vi "UI (Beginner).vi"() -> ()   [LabVIEW 2017, in "UI.lvlib"]
doc: "The Queued Message Handler of a Worker."
uses:
  UI.lvlib
  _support/UI State.ctl
  1af51285-6659-428e-9c15-de70f1a207c9.vi
  1756710f-d813-4077-a3f9-6f06171a4225.vi
  b1498353-a107-4479-98d0-7e76c0451ff6.vi
  242d01f8-d211-4c25-bb6c-8191a2acbe42.vi
  <userlib>/_NEVSTOP/Communicable State Machine(CSM)/AdvanceAPI/CSM - Revert Arguments-Safe String.vi
  <userlib>/_NEVSTOP/Communicable State Machine(CSM)/_Shared/Trim Single-line Text.vi
  <userlib>/_NEVSTOP/Communicable State Machine(CSM)/AdvanceAPI/CSM - Make String Arguments Safe.vi
  <userlib>/_NEVSTOP/Communicable State Machine(CSM)/AdvanceAPI/CSM - Break Down Multiple States String.vi
  <userlib>/_NEVSTOP/Communicable State Machine(CSM)/AdvanceAPI/CSM - Keywords.vi
  <userlib>/_NEVSTOP/Communicable State Machine(CSM)/addons/INI-Static-Variable-Support/_Support/instances/_CSM - Read File Logger Configuration - v1.0.vi
  <userlib>/_NEVSTOP/Communicable State Machine(CSM)/addons/API-String-Arugments-Support/_Support/Convert API String Arguments to Data(variant).vi
  <userlib>/_NEVSTOP/Communicable State Machine(CSM)/addons/API-String-Arugments-Support/_Support/Query Data as API String Arguments(variant).vi
  <userlib>/_NEVSTOP/Communicable State Machine(CSM)/addons/MassData-Parameter/_support/FGV-MassData(lvlibp).vi
  <userlib>/_NEVSTOP/Communicable State Machine(CSM)/_Polymophic/Add State(s) to Queue By BOOL(Element).vi
  Acquisition/Acquisition.lvlib
  Logging/Logging.lvlib
  <userlib>/_NEVSTOP/Communicable State Machine(CSM)/Communicable State Machine.lvlib
  <userlib>/_NEVSTOP/Communicable State Machine(CSM)/addons/MassData-Parameter/CSM MassData Parameter Support.lvlib
  <userlib>/_NEVSTOP/Communicable State Machine(CSM)/addons/INI-Static-Variable-Support/INI-Static-Variable-Support.lvlib
  <userlib>/_NEVSTOP/Communicable State Machine(CSM)/addons/Logger/CSM File Logger.lvlib
  <userlib>/_NEVSTOP/Communicable State Machine(CSM)/addons/Watchdog/CSM Watchdog.lvlib
  <userlib>/_NEVSTOP/Communicable State Machine(CSM)/_Polymophic/Build Synchronous Message with Arguments.vi
panel:
  out "WaveformGraph":waveform(dbl)[](graph)
  in  "Settings":bool
  in  "Start":bool
  in  "Stop":bool
  out "Status":string
  in  "Exit":bool
  # "Continuous Measurement and Data Logger - CSM Version"
  # "Beginner Example"
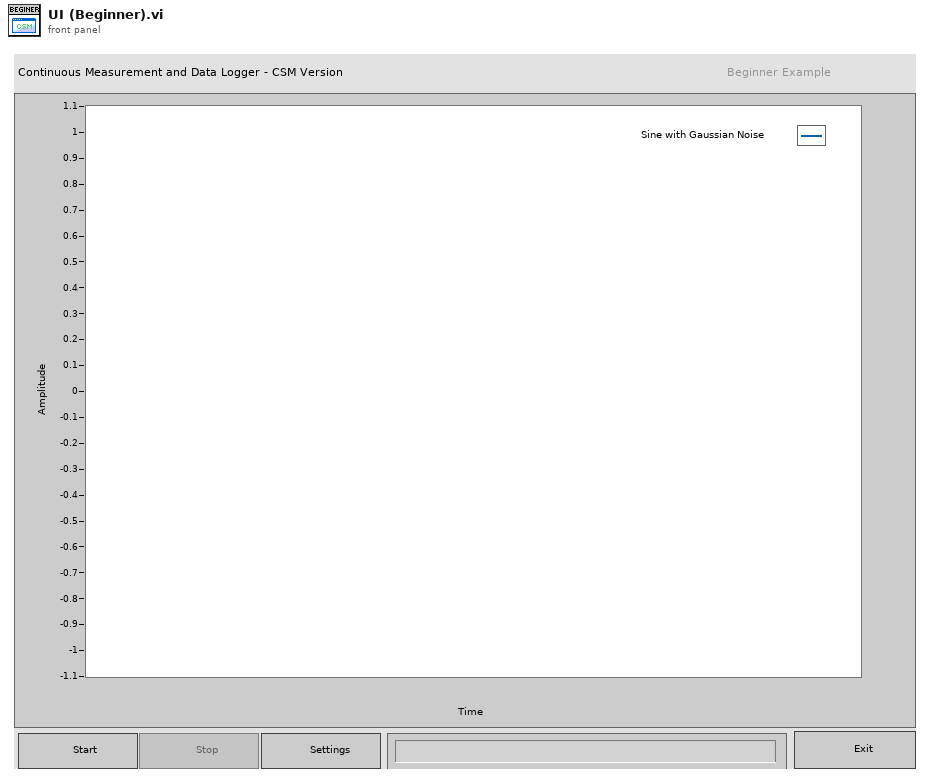
[diagram p1: front panel]
types:
  T1 = cluster{"Enable":bool, "Limit":cluster{"FileSize":i64, "FileNum":i32}, "Timestamp.Format":string, "AutoExit":bool}
  T2 = enum32{"Invalid", "Standard", "Closed", "Hidden", "Minimized", "Maximized"}
  T3 = enum32{"invalid app kind", "Development System", "Run Time System", "Student Edition", "Embedded LabVIEW", "Evaluation", "Custom"}
  T4 = typedef "UI.lvlib/UI State.ctl" = enum16{"Idle", "Acquiring and Logging", "Waiting for Exit", "Waiting for Exit (Acq Stopped)", "Waiting for Exit (Log Stopped)", "Waiting for Stop", "Waiting for Stop (Acq Stopped)", "Waiting for Stop (Log Stopped)"}
  T5 = enum32{"Invalid", "Default", "Floating", "Floating/Auto-Hide", "Modal"}
  T6 = typedef "Communicable State Machine.lvlib/_CSM_Response Source Message.ctl" = cluster{"‘State":string, "’Arguments":string, "’Error":errorcluster}
  T7 = cluster{"Current VI Reference":refnum<vi>, "Close Panel on Exit?":bool}
  T8 = cluster{"Core":cluster{"Current VI Reference":refnum<vi>, "Close Panel on Exit?":bool}, "UI Refs":cluster{"Start Ref":refnum<vi>, "Stop Ref":refnum<vi>, "Settings Ref":refnum<vi>, "Exit Ref":refnum<vi>, "Status Ref":refnum<vi>, "Data Ref":refnum<vi>, "Data Source Ref":refnum<vi>}, "State":T4, "Relationships":string}
  T9 = cluster{"Start Ref":refnum<vi>, "Stop Ref":refnum<vi>, "Settings Ref":refnum<vi>, "Exit Ref":refnum<vi>, "Status Ref":refnum<vi>, "Data Ref":refnum<vi>, "Data Source Ref":refnum<vi>}
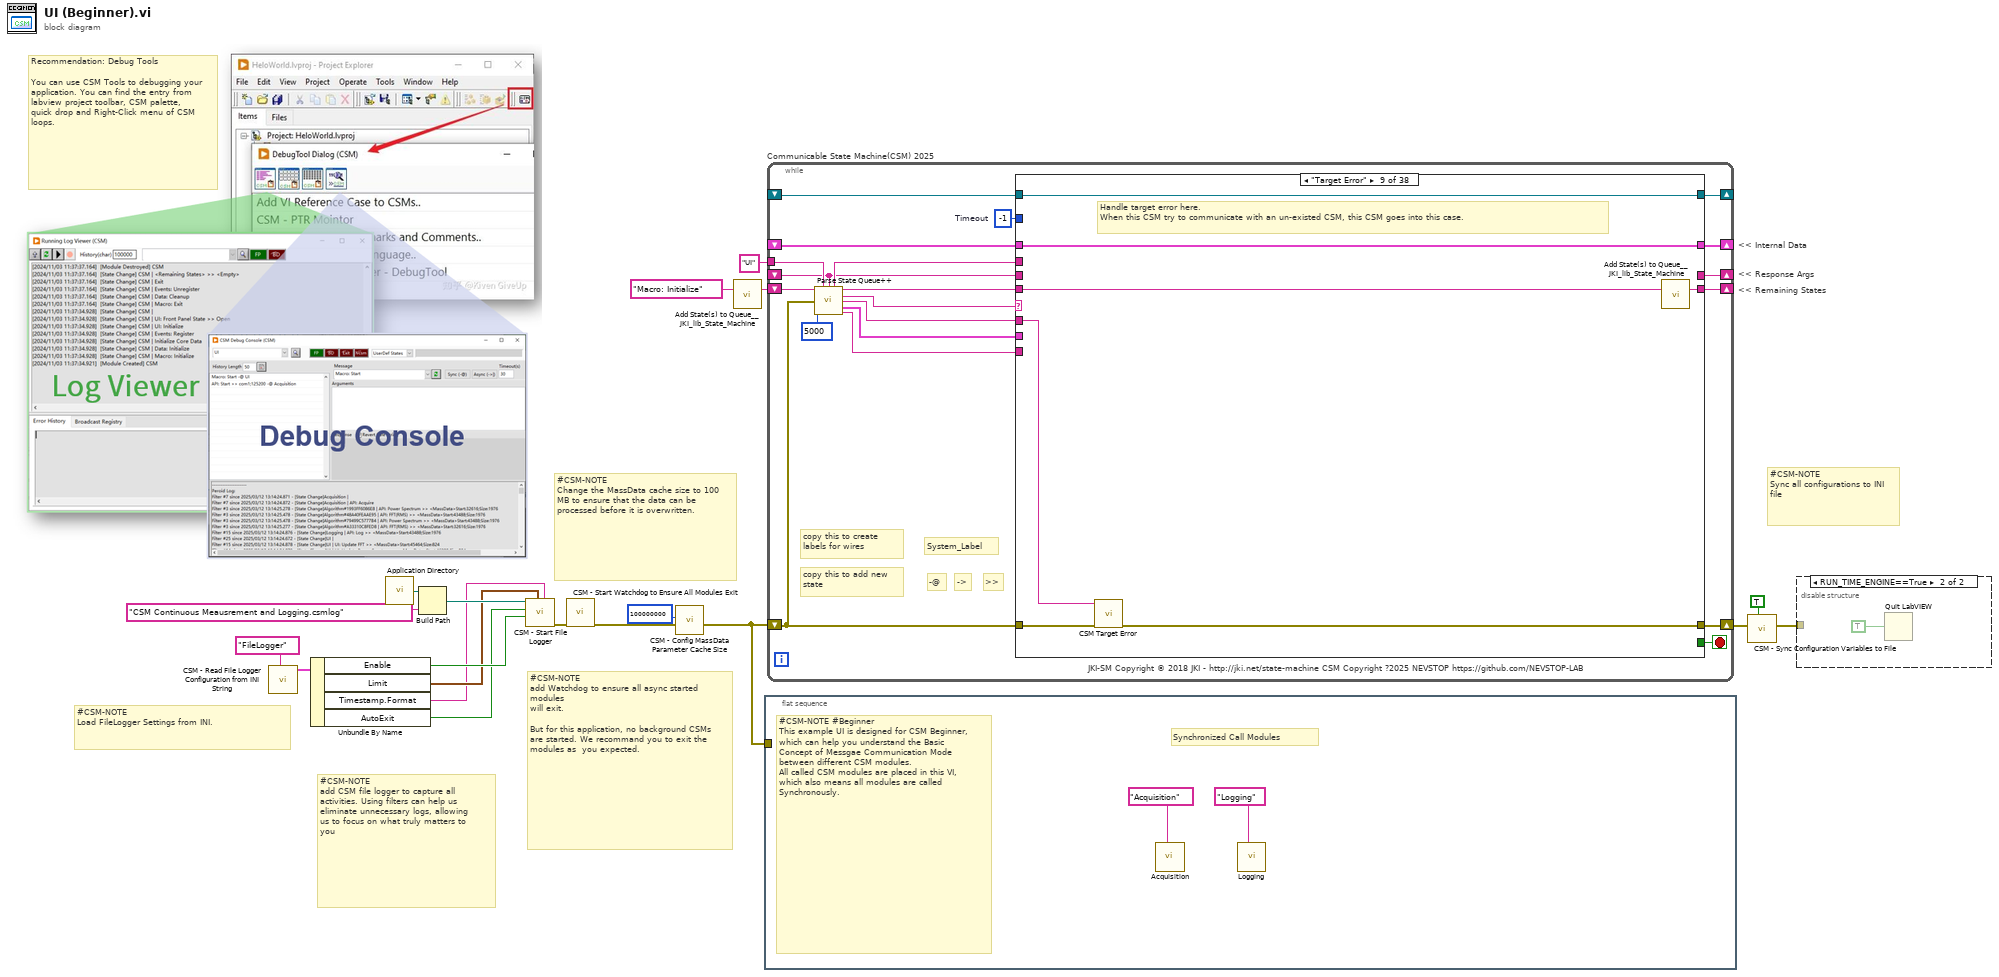
[diagram p0: block diagram]
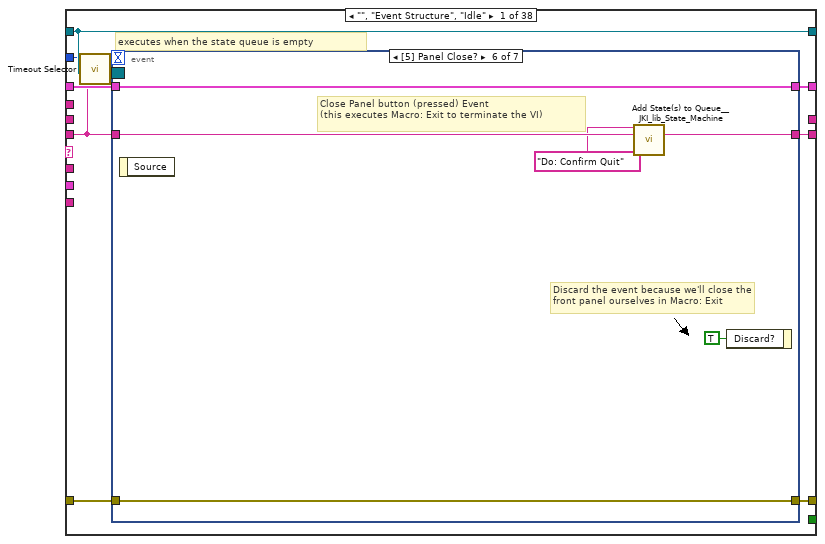
[diagram p3: hidden frame]
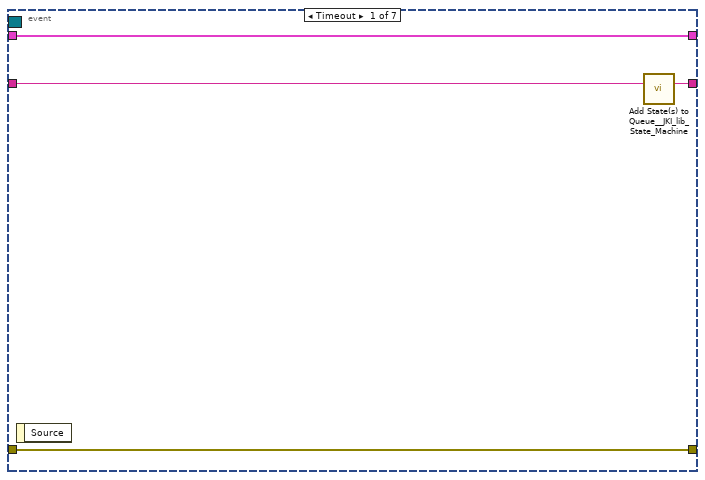
[diagram p4: hidden frame]
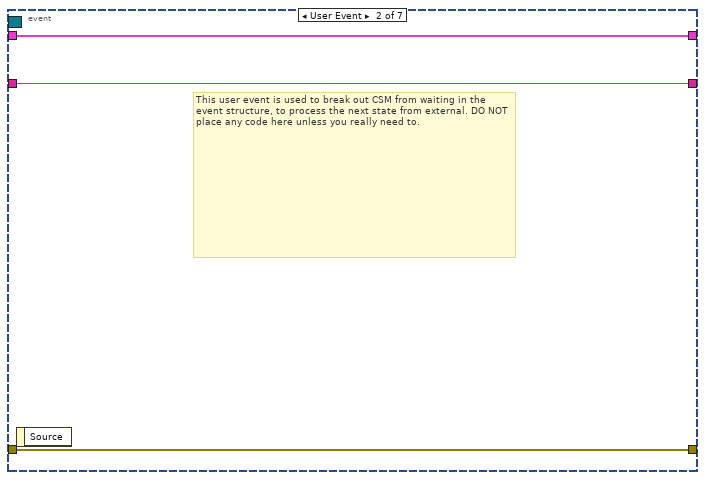
[diagram p5: hidden frame]
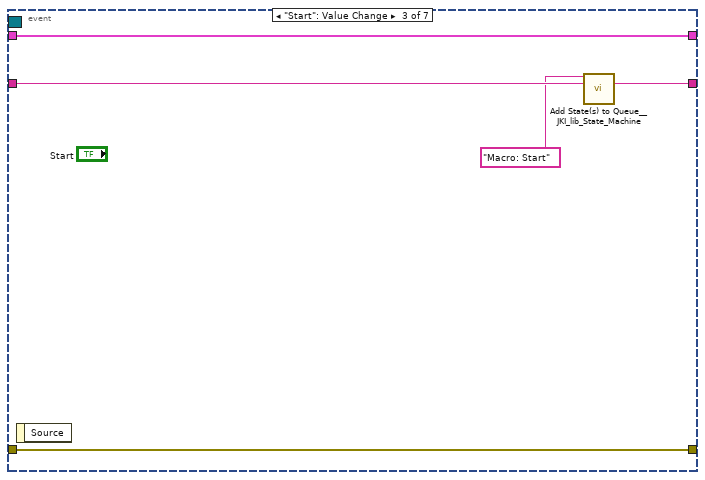
[diagram p6: hidden frame]
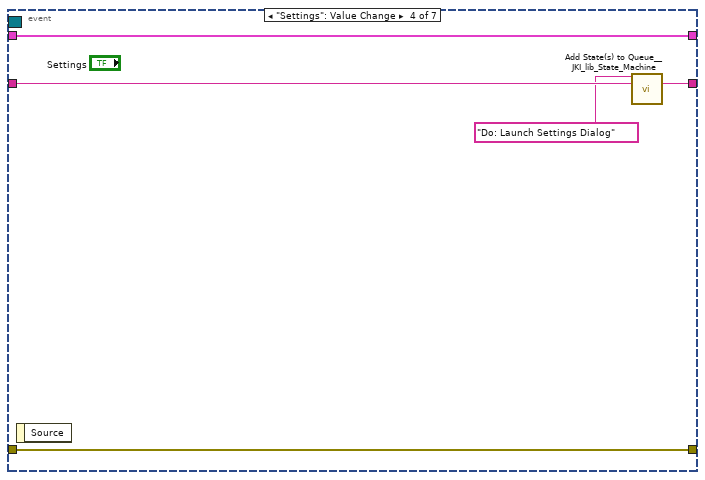
[diagram p7: hidden frame]
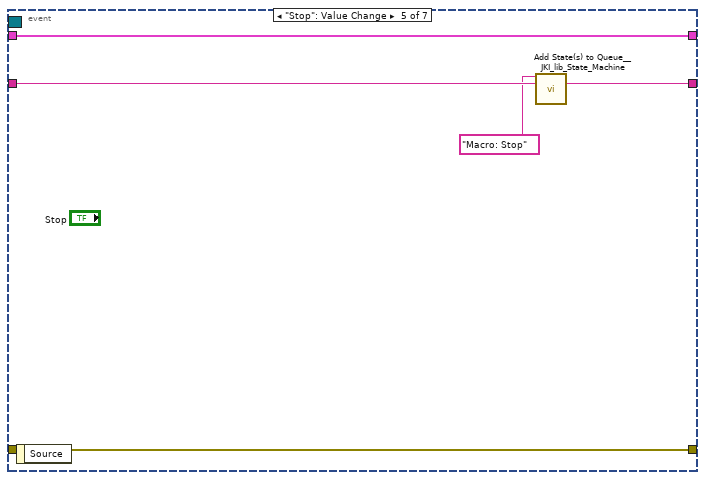
[diagram p8: hidden frame]
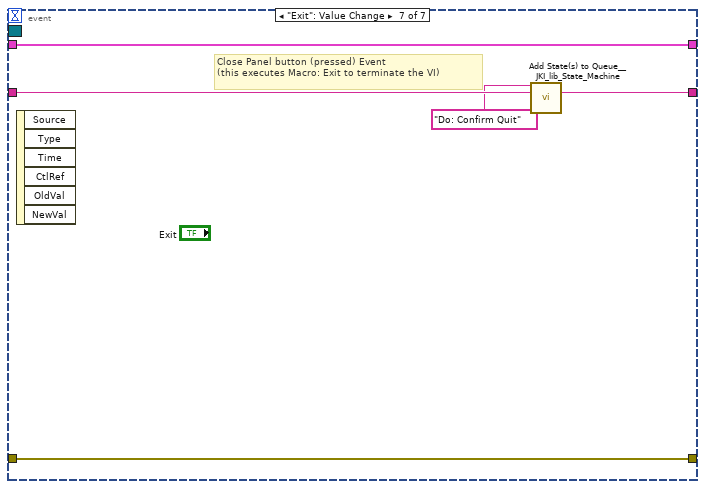
[diagram p9: hidden frame]
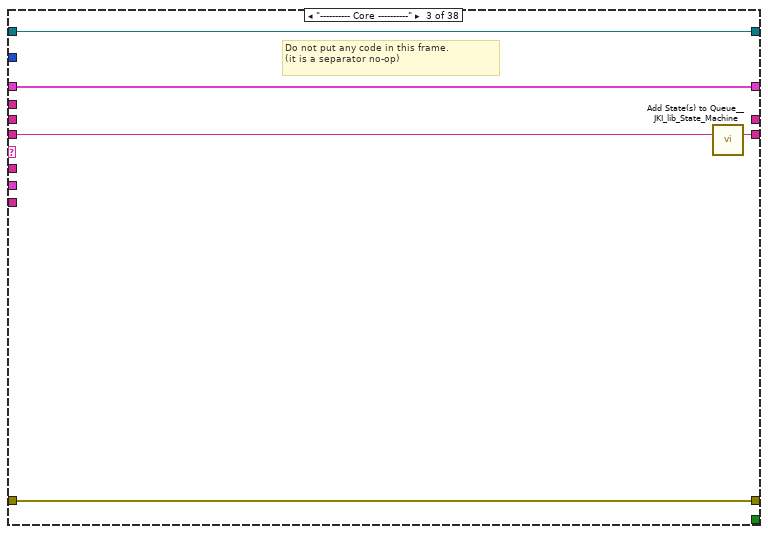
[diagram p11: hidden frame]
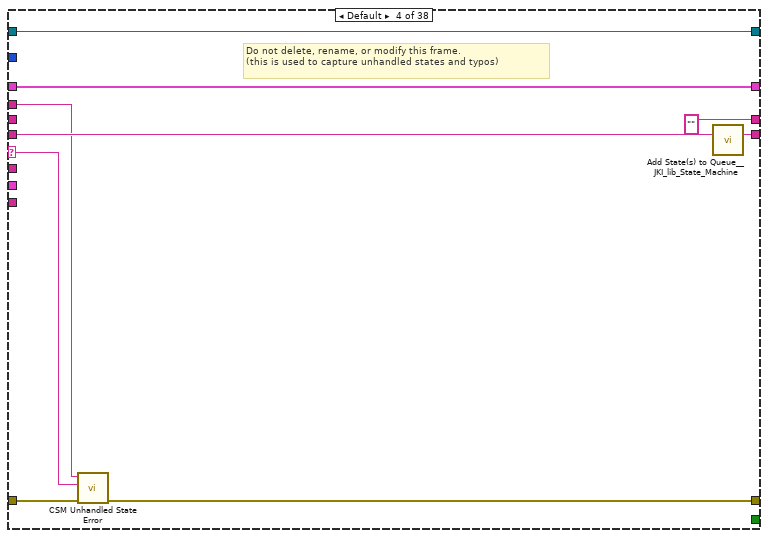
[diagram p12: hidden frame]
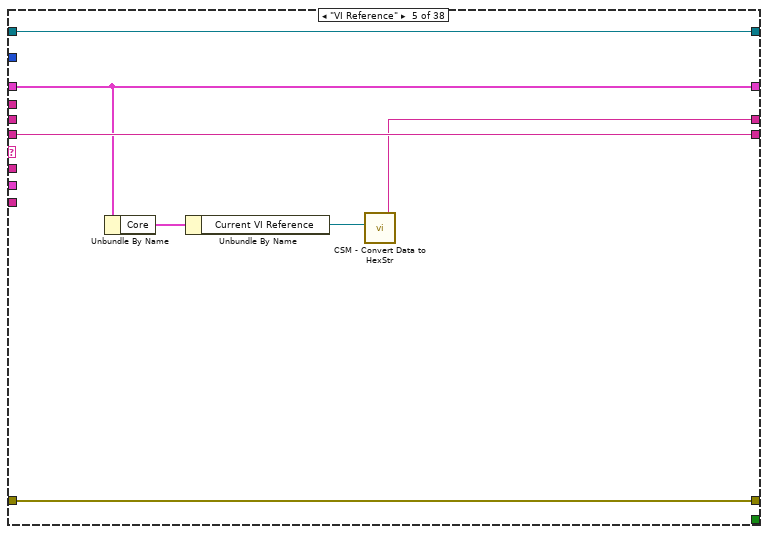
[diagram p13: hidden frame]
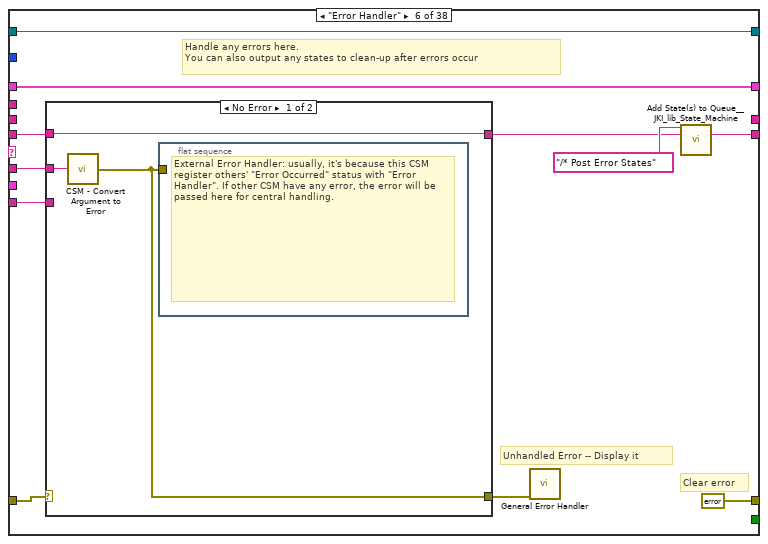
[diagram p14: hidden frame]
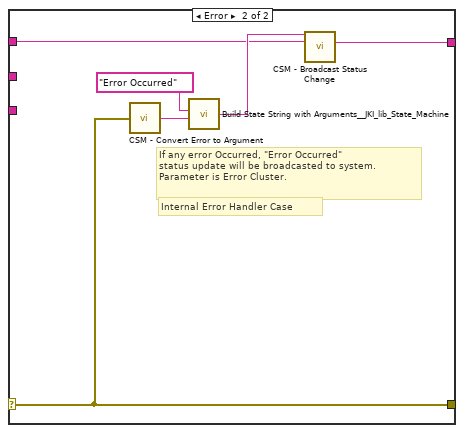
[diagram p15: hidden frame]
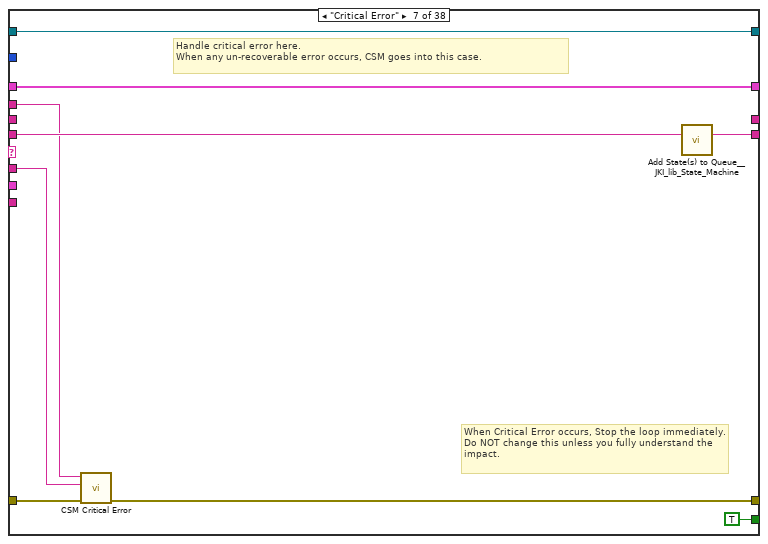
[diagram p16: hidden frame]
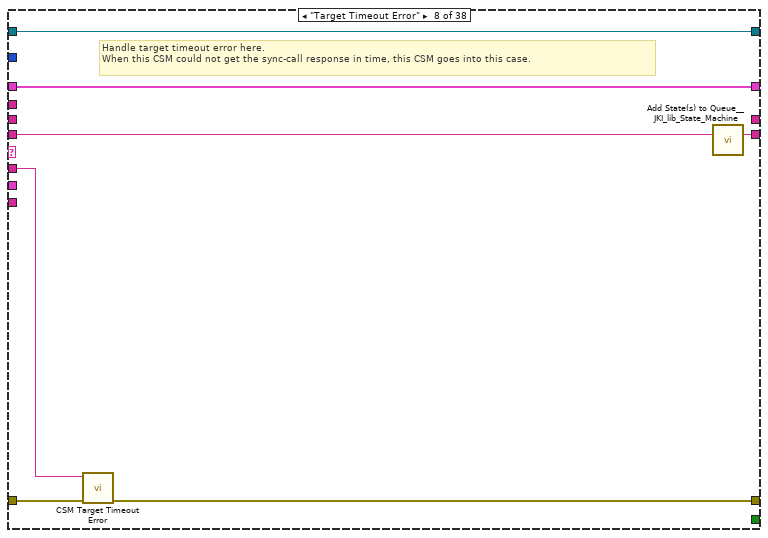
[diagram p17: hidden frame]
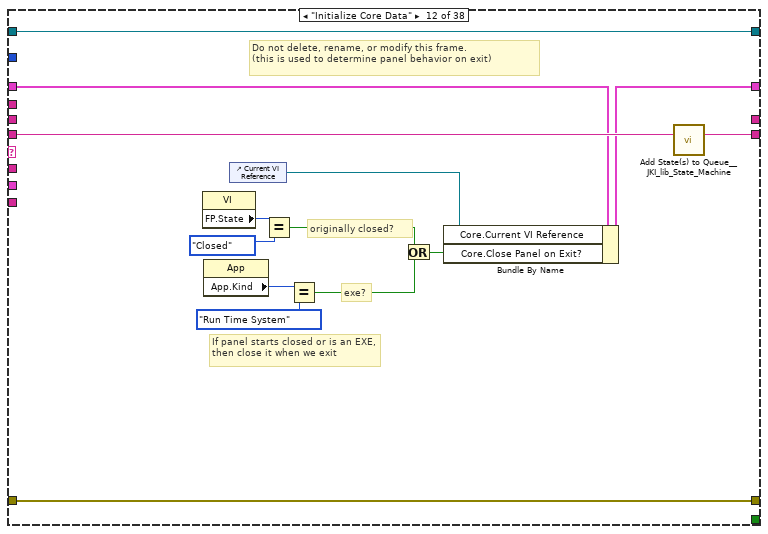
[diagram p20: hidden frame]
diagram:
  # "#CSM-NOTE\nSync all configurations to INI file"
  # "#CSM-NOTE\nChange the MassData cache size to 100 MB to ensure that the data can be processed before it is overwritten."
  # "Recommendation: Debug Tools\n\nYou can use CSM Tools to debugging your application. You can find the entry from labview project toolbar, CSM palette, quick drop and Right-Click menu of CSM loops."
  # "#CSM-NOTE\nLoad FileLogger Settings from INI."
  # "#CSM-NOTE\nadd CSM file logger to capture all activities. Using filters can help us eliminate unnecessary logs, allowing us to focus on what truly matters to you"
  # "#CSM-NOTE\nadd Watchdog to ensure all async started modules\nwill exit. \n\nBut for this application, no background CSMs are started. We recommand you to exit the modules as  you expected."
  # "<< Internal Data"
  # "<< Response Args"
  # "<< Remaining States"
  n1 = call-poly <userlib>:"CSM - Read File Logger Configuration from INI String.vi"("Section Name(\"FileLogger\")"="FileLogger" ("Section Name(\"\" as Default)")) -> ("FileLogger Configuration-v1"=w11:T1)  [unwired: 7 in, 1 out]
  n2 = Unbundle By Name(w11) -> ("Enable"=w10:bool, "Limit"=w9:cluster{"FileSize":i64, "FileNum":i32}, "Timestamp.Format"=w7:string, "AutoExit"=w8:bool)
  n3 = call <vilib>:"Application Directory.vi"() -> ("Application Directory"=w16:path)
  n4 = Build Path(base path=w16, name or relative path="CSM Continuous Meausrement and Logging.csmlog") -> (appended path=w14:path)
  n5 = call <userlib>:"CSM - Start File Logger.vi"("Timestamp Format"=w7, "Log Limit"=w9, "Watchdog? (T)"=w10, "Exit When All Module Exist? (F)"=w8, "Log File Path"=w14) -> ("error out"=w13:errorcluster)  [unwired: 4 in, 2 out]
  n6 = call <userlib>:"CSM - Start Watchdog to Ensure All Modules Exit.vi"("error in (no error)"=w13) -> ("error out"=w5:errorcluster)  [unwired: 10 in]
  n7 = call <userlib>:"CSM - Config MassData Parameter Cache Size.vi"("Error in"=w5, "Size (50M)"=100000000 ("size(1M)")) -> ("Error out"=w4:errorcluster)  [unwired: 9 in]
  n8 = call <vilib>:"Add State(s) to Queue__JKI_lib_State_Machine.vi"("State(s) in (\"\")"="Macro: Initialize") -> ("States Out"=w17:string)  [unwired: 14 in]
  n9 = flat-sequence {
    tunnel: w4 -> [_]
    frame #0 {
      # "Synchronized Call Modules"
      # "#CSM-NOTE #Beginner\nThis example UI is designed for CSM Beginner, which can help you understand the Basic Concept of Messgae Communication Mode between different CSM modules.\nAll called CSM modules are placed in this VI, which also means all modules are called  Synchronously."
      n10 = call "Acquisition.vi"("Name(\"\" to use uuid)"="Acquisition" ("Name(\"\" to use uuid)")) -> ()  [unwired: 11 in]
      n11 = call "Logging.vi"("Name(\"\" to use uuid)"="Logging" ("Name(\"\" to use uuid)")) -> ()  [unwired: 11 in]
    }
  }
  n12 = while "Communicable State Machine(CSM) 2025" {
    shift-right: [w36] -> _
    shift-left: _ -> [w35]
    shift-right: [w39] -> w2
    shift-left: w4 -> [w33]
    shift-right: [w38] -> _
    shift-left: w17 -> [w40]
    tunnel: "UI" ("Name(\"\" to use uuid)") -> [w28]
    shift-right: [w31] -> _
    shift-left: _ -> [w23]
    shift-right: [w30] -> _
    shift-left: _ -> [w29]
    stop <- w37 stop-if-true
    w34 = -1  # Timeout
    # "JKI-SM Copyright © 2018 JKI - http://jki.net/state-machine CSM Copyright ?2025 NEVSTOP https://github.com/NEVSTOP-LAB"
    # "copy this to add new state"
    # ">>"
    # "->"
    # "-@"
    # "copy this to create labels for wires"
    # "System_Label"
    n13 = call <userlib>:"Parse State Queue++.vi"("State Queue"=w40, "Name (\"\" to Use UUID)"=w28, "Response Arguments"=w23, "Previous Error"=w33, "Response Timeout (-2 Use Global Settings)"=5000 ("Response Timeout(1000ms)")) -> ("Name Used"=w24:string, "Remaining States"=w41:string, "Current State"=w27:string, "Arguments"=w22:string, "Additional Information"=w26:T6, "Source CSM"=w25:string)  [unwired: 5 in]
    n14 = case shown="\"Target Error\"" w27 {
      selector: w27 -> [_ _ _ w95 _ _ _ _ _ _ _ _ _ _ _ _ _ _ _ _ _ _ _ _ _ _ _ _ _ _ _ _ _ _ _ _ _ _]
      tunnel: w41 -> [w42 w86 w92 w100 w107 w112 w135 w143 w150 w154 w158 w173 w180 w185 w194 w200 w207 w214 w219 w225 w229 w235 w252 w265 w278 w286 w302 w376 w385 w396 w403 w405 w416 w434 w459 w465 w473 w511]
      tunnel: w22 -> [_ _ _ _ _ w110 w129 w139 w146 _ _ _ _ _ _ w198 w204 _ _ _ _ _ _ _ _ w281 w296 w371 w389 _ _ _ _ _ _ w460 _ _]
      tunnel: w35 -> [w49 w85 w89 w98 w106 w118 w136 w141 w148 w153 w157 w166 w178 w182 _ w197 w205 w209 w216 w224 w228 w232 w239 w255 w268 w284 w298 w374 w391 w393 w400 w408 w412 w432 w456 w462 w466 w506]
      tunnel: [w48 w87 w90 w94 w108 errorcluster {"status"=FALSE, "code"=0, "source"=""} ("error out") w131 w138 w145 w155 w159 w170 w177 w183 w188 w196 w203 w210 w217 w220 w227 w233 w250 w266 w279 w282 w299 w368 w387 w394 w401 w411 w420 _ w457 w463 w467 _] -> w39
      tunnel: w33 -> [w47 w87 w90 w101 w108 w116 w137 w144 w151 w155 w159 w170 w177 w183 w188 _ _ w211 w217 _ w230 w233 w250 w266 w279 w283 w300 _ _ w394 w401 w411 w420 _ w457 w463 _ _]
      tunnel: [w50 w86 w91 w99 w107 w114 w134 w142 w149 w154 w158 w172 w179 w184 w193 w200 w207 w213 w218 w225 w229 w234 w251 w265 w278 w285 w301 w376 w386 w395 w402 w406 w417 w433 w458 w464 w473 w504] -> w38
      tunnel: [_ _ _ _ _ _ TRUE _ _ _ _ _ TRUE _ _ _ _ _ _ _ _ _ _ _ _ _ _ _ _ _ _ _ _ _ _ _ _ _] -> w37
      tunnel: [w46 w85 w89 w98 w106 w118 w136 w141 w148 w153 w157 w171 w178 w182 w187 w195 w201 w209 w216 w224 w228 w232 w238 w255 w268 w284 w298 w374 w391 w393 w400 w407 w418 w432 w456 w462 w466 w505] -> w36
      tunnel: w34 -> [w44 _ _ _ _ _ _ _ _ _ _ _ _ _ _ _ _ _ _ _ _ _ _ _ _ _ _ _ _ _ _ _ _ _ _ _ _ _]
      tunnel: w25 -> [_ _ _ _ _ w109 _ _ _ _ _ _ _ _ _ _ _ _ _ _ _ _ _ _ _ _ _ _ _ _ _ _ _ _ _ _ _ _]
      tunnel: w26 -> [_ _ _ _ _ _ _ _ _ _ _ _ _ _ _ _ _ _ _ _ _ _ _ _ _ _ _ _ _ _ _ _ _ _ _ _ _ _]
      tunnel: [_ _ _ "" w102 _ _ _ _ _ _ _ _ _ _ _ w202 _ _ _ _ _ _ _ _ _ _ _ _ _ _ _ _ _ _ _ _ _] -> w31
      tunnel: [w45 w84 w88 w96 w105 w117 w132 w140 w147 w152 w156 w160 w175 w181 w191 w199 w206 w208 w215 w223 w226 w231 w249 w264 w277 w280 w295 w375 w390 w392 w399 w410 w419 w425 w455 w461 w474 w510] -> w30
      tunnel: w29 -> [w45 w84 w88 w96 w105 w117 w132 w140 w147 w152 w156 w160 w175 w181 w191 w199 w206 w208 w215 _ w226 w231 w249 w264 w277 w280 w295 w375 w390 w392 w399 w410 w419 w425 w455 w461 w474 w510]
      tunnel: w24 -> [_ _ _ w93 _ _ w130 _ _ _ _ _ _ _ _ _ _ _ _ w222 _ _ _ _ _ _ _ _ _ _ _ _ _ w423 _ _ w469 _]
      tunnel: w23 -> [_ _ _ _ _ _ _ _ _ _ _ _ _ _ _ _ _ _ _ _ _ _ _ _ _ _ _ _ _ _ _ _ _ _ _ _ _ _]
      frame "", "Event Structure", "Idle" {
        # "executes when the state queue is empty"
        n15 = call <userlib>:"Timeout Selector.vi"("Remaining States"=w42, "Timeout Expected"=w44) -> ("Timeout"=w43:i32)  [unwired: 5 in]
        n16 = event shown="[5] Panel Close?" {
          selector: w45 -> [_ _ _ _ _ _ _]
          dyn-events: _ -> [_ _ _ _ _ _ _]
          timeout: w43 -> [_ _ _ _ _ _ _]
          tunnel: w42 -> [w54 w56 w59 w64 w69 w78 w83]
          tunnel: [w53 w56 w60 w65 w70 w77 w82] -> w50
          tunnel: w49 -> [w51 w57 w61 w66 w71 w75 w80]
          tunnel: [w52 w55 w62 w67 w72 w76 w81] -> w48
          tunnel: w47 -> [w52 w55 w62 w67 w72 w76 w81]
          tunnel: [w51 w57 w61 w66 w71 w75 w80] -> w46
          event Timeout {
            n17 = event-data() -> ()  [unwired: 1 in, 1 out]
            n18 = call <vilib>:"Add State(s) to Queue__JKI_lib_State_Machine.vi"("State(s) in (\"\")"=w54) -> ("States Out"=w53:string)  [unwired: 14 in]
          }
          event User Event {
            # "This user event is used to break out CSM from waiting in the event structure, to process the next state from external. DO NOT place any code here unless you really need to."
            n19 = event-data() -> ()  [unwired: 1 in, 1 out]
          }
          event "Start": Value Change {
            n20 = event-data() -> ()  [unwired: 1 in, 1 out]
            n21 = call <vilib>:"Add State(s) to Queue__JKI_lib_State_Machine.vi"("State(s) in Front (\"\")"="Macro: Start" ("State(s) in Front (\"\")"), "State(s) in (\"\")"=w59) -> ("States Out"=w60:string)  [unwired: 13 in]
          }
          event "Settings": Value Change {
            n22 = event-data() -> ()  [unwired: 1 in, 1 out]
            n23 = call <vilib>:"Add State(s) to Queue__JKI_lib_State_Machine.vi"("State(s) in Front (\"\")"="Do: Launch Settings Dialog" ("State(s) in Front (\"\")"), "State(s) in (\"\")"=w64) -> ("States Out"=w65:string)  [unwired: 13 in]
          }
          event "Stop": Value Change {
            n24 = event-data() -> ()  [unwired: 1 in, 1 out]
            n25 = call <vilib>:"Add State(s) to Queue__JKI_lib_State_Machine.vi"("State(s) in Front (\"\")"="Macro: Stop" ("State(s) in Front (\"\")"), "State(s) in (\"\")"=w69) -> ("States Out"=w70:string)  [unwired: 13 in]
          }
          event Panel Close? {
            # "Discard the event because we'll close the front panel ourselves in Macro: Exit"
            # "Close Panel button (pressed) Event\n(this executes Macro: Exit to terminate the VI)"
            n26 = event-data() -> ()  [unwired: 1 in, 1 out]
            n27 = call <vilib>:"Add State(s) to Queue__JKI_lib_State_Machine.vi"("State(s) in Front (\"\")"="Do: Confirm Quit", "State(s) in (\"\")"=w78) -> ("States Out"=w77:string)  [unwired: 13 in]
            n28 = event-data("Discard?"=TRUE) -> ()  [unwired: 1 in, 1 out]
          }
          event "Exit": Value Change {
            # "Close Panel button (pressed) Event\n(this executes Macro: Exit to terminate the VI)"
            n29 = event-data() -> ()  [unwired: 1 in, 6 out]
            n30 = call <vilib>:"Add State(s) to Queue__JKI_lib_State_Machine.vi"("State(s) in Front (\"\")"="Do: Confirm Quit", "State(s) in (\"\")"=w83) -> ("States Out"=w82:string)  [unwired: 13 in]
          }
        }
      }
      frame "CSM Documentation" {
        # "CSM Documentation"
        # "State Syntax:\nStateCategory: State >> Argument -@ CSMName\nStateCategory: State >> Argument -> CSMName\n\nLine Terminator: Line feed"
        # "Commenting:\nTo add a comment use \"//\" or \"#\" and all text to the right will be ignored\nCommenting Example:\nUI: Initialize // This initializes the UI\n// Another comment line"
        # "Example:\nUI: Help >> About -@Main\nUI: Help >> About ->Main\n\nWhere \"UI\" is the state category\nWhere \"Help\" is the state\nWhere \"About\" is the argument\nWhere \"Main\" is the Name of CSM,which actually run the \"UI: Help >> About\"\n\n    \"-@\" stands for sync state. Current CSM will wait until the state is finished. \n            - if \"Main\" named CSM does not exist, \"Target Error\" will occur.\n            - if \"Main\" named CSM is in another sync remote state, \"Target Busy Error\" will occur.\n            - if \"Main\" named CSM could not finish the state in time, \"Target Timeout Error\" will occur.\n            - if everything is right. \"Response\" will occur with Argument back from \"Main\" named CSM. \n\n    \"->\" stands for async state. Current CSM will post the state and continue to next state in next iteration.\n            - if \"Main\" named CSM does not exist, \"Target Error\" will occur.\n            - if everything is right. \"Async Message Posted\" will occur.\n            - After State is finished. Caller will receive a \"Async Response\" state from callee.\n\nWhen duplicated name is used for multiple CSM module or some framework problem happens, \"Critical Error\" will occur."
      }
      frame "---------- Core ----------" {
        # "Do not put any code in this frame.\n(it is a separator no-op)"
        n31 = call <vilib>:"Add State(s) to Queue__JKI_lib_State_Machine.vi"("State(s) in (\"\")"=w92) -> ("States Out"=w91:string)  [unwired: 14 in]
      }
      frame Default {
        # "Do not delete, rename, or modify this frame.\n(this is used to capture unhandled states and typos)"
        n32 = call <userlib>:"CSM Unhandled State Error.vi"("error in (no error)"=w101, "Undefined State"=w95, "CSM Name"=w93) -> ("error out"=w94:errorcluster)  [unwired: 8 in]
        n33 = call <vilib>:"Add State(s) to Queue__JKI_lib_State_Machine.vi"("State(s) in (\"\")"=w100) -> ("States Out"=w99:string)  [unwired: 14 in]
      }
      frame "VI Reference" {
        n34 = Unbundle By Name(w106) -> ("Core"=w104:T7)
        n35 = Unbundle By Name(w104) -> ("Current VI Reference"=w103:refnum<vi>)
        n36 = call <userlib>:"CSM - Convert Data to HexStr.vi"("Variant"=w103) -> ("HEX String (0-9,A-F)"=w102:string)  [unwired: 8 in]
      }
      frame "Error Handler" {
        # "Unhandled Error -- Display it"
        # "Handle any errors here.\nYou can also output any states to clean-up after errors occur"
        # "Clear error"
        n37 = case shown="No Error" w116 {
          selector: w116 -> [_ w123]
          tunnel: [w121 w125] -> w113
          tunnel: w112 -> [w121 w124]
          tunnel: [w120 w123] -> w111
          tunnel: w110 -> [w122 _]
          tunnel: w109 -> [_ _]
          frame No Error {
            n38 = call <userlib>:"CSM - Convert Argument to Error.vi"("Argument"=w122) -> ("Error"=w120:errorcluster)  [unwired: 4 in]
            n39 = flat-sequence {
              tunnel: w120 -> [_]
              frame #0 {
                # "External Error Handler: usually, it's because this CSM register others' \"Error Occurred\" status with \"Error Handler\". If other CSM have any error, the error will be passed here for central handling."
              }
            }
          }
          frame Error {
            # "Internal Error Handler Case"
            # "If any error Occurred, \"Error Occurred\" \nstatus update will be broadcasted to system.\nParameter is Error Cluster."
            n40 = call <userlib>:"CSM - Convert Error to Argument.vi"("Error"=w123) -> ("Argument"=w127:string)  [unwired: 4 in]
            n41 = call <vilib>:"Build State String with Arguments__JKI_lib_State_Machine.vi"("Arguments (\"\")"=w127, "State"="Error Occurred" ("Status with Arguments")) -> ("State with Arguments"=w126:string)  [unwired: 4 in]
            n42 = call <userlib>:"CSM - Broadcast Status Change.vi"("Status With Arguments"=w126, "State Queue"=w124) -> ("Remaining States"=w125:string)  [unwired: 13 in]
          }
        }
        n43 = call <vilib>:"General Error Handler.vi"("error in (no error)"=w111) -> ()  [unwired: 10 in, 5 out]
        n44 = call <vilib>:"Add State(s) to Queue__JKI_lib_State_Machine.vi"("State(s) in Front (\"\")"="/* Post Error States", "State(s) in (\"\")"=w113) -> ("States Out"=w114:string)  [unwired: 13 in]
      }
      frame "Critical Error" {
        # "Handle critical error here.\nWhen any un-recoverable error occurs, CSM goes into this case."
        # "When Critical Error occurs, Stop the loop immediately. Do NOT change this unless you fully understand the impact."
        n45 = call <userlib>:"CSM Critical Error.vi"("error in (no error)"=w137, "Arugments (As Reason)"=w129, "CSM Name"=w130) -> ("error out"=w131:errorcluster)  [unwired: 8 in]
        n46 = call <vilib>:"Add State(s) to Queue__JKI_lib_State_Machine.vi"("State(s) in (\"\")"=w135) -> ("States Out"=w134:string)  [unwired: 14 in]
      }
      frame "Target Timeout Error" {
        # "Handle target timeout error here.\nWhen this CSM could not get the sync-call response in time, this CSM goes into this case."
        n47 = call <userlib>:"CSM Target Timeout Error.vi"("error in (no error)"=w144, "Arguments (As CSM Name)"=w139) -> ("error out"=w138:errorcluster)  [unwired: 9 in]
        n48 = call <vilib>:"Add State(s) to Queue__JKI_lib_State_Machine.vi"("State(s) in (\"\")"=w143) -> ("States Out"=w142:string)  [unwired: 14 in]
      }
      frame "Target Error" {
        # "Handle target error here.\nWhen this CSM try to communicate with an un-existed CSM, this CSM goes into this case."
        n49 = call <userlib>:"CSM Target Error.vi"("error in (no error)"=w151, "Arguments (As CSM Name)"=w146) -> ("error out"=w145:errorcluster)  [unwired: 9 in]
        n50 = call <vilib>:"Add State(s) to Queue__JKI_lib_State_Machine.vi"("State(s) in (\"\")"=w150) -> ("States Out"=w149:string)  [unwired: 14 in]
      }
      frame "Async Response", "Response" {
        # "Handle Async-call Response (\"Async Response\" for ->)"
        # "Handle Sync-call Response (\"Response\" for -@)"
        # "After Message is executed, CSM+ goes to this state for receive the response. \n    For Async Message(->), \"Async Response\" is used. This CSM will goes to \"Async Message Posted\" immediately and receive the \"Async Response\" after the callee finishes the message.\n    For Sync Message(@),  This CSM will wait until the message is done and immediately goes to \"Response\""
      }
      frame "Async Message Posted" {
        # "Handle post action for async message (->)."
        # "After Async Message is posted (->), CSM+ goes to this state for post-action. You can use Argument - State to tell which Async Message is called."
      }
      frame "Initialize Core Data" {
        # "Do not delete, rename, or modify this frame.\n(this is used to determine panel behavior on exit)"
        # "originally closed?"
        # "exe?"
        # "If panel starts closed or is an EXE, then close it when we exit"
        n51 = property class="VI"() -> ("FP.State"=w163:T2)  [unwired: 2 in, 2 out]
        n52 = property class="App"() -> ("App.Kind"=w169:T3)  [unwired: 2 in, 2 out]
        n53 = control-ref of="Current VI Reference"() -> (w164:refnum<vi>)
        n54 = Equal?(x=w163, y=T2."Closed" ("Front Panel Window:State")) -> (x = y?=w161:bool)
        n55 = Equal?(x=w169, y=T3."Run Time System" ("Application:Kind")) -> (x = y?=w167:bool)
        n56 = Or(x=w161, y=w167) -> (x .or. y?=w165:bool)
        n57 = Bundle By Name(cluster=w166, "Core.Current VI Reference"=w164, "Core.Close Panel on Exit?"=w165) -> (w171:T8)
        n58 = call <vilib>:"Add State(s) to Queue__JKI_lib_State_Machine.vi"("State(s) in (\"\")"=w173) -> ("States Out"=w172:string)  [unwired: 14 in]
      }
      frame "Exit" {
        # "Do not put any code in this frame.\n(No errors that occur here will be handled.)"
        n59 = local write "Status"("Exit" ("Exit String")) -> ()
        n60 = call <vilib>:"Add State(s) to Queue__JKI_lib_State_Machine.vi"("State(s) in (\"\")"=w180) -> ("States Out"=w179:string)  [unwired: 14 in]
      }
      frame "---------- Data ----------" {
        # "Do not put any code in this frame.\n(It is a separator no-op. You can make a copy of this frame to create a new Data frame)"
        n61 = call <vilib>:"Add State(s) to Queue__JKI_lib_State_Machine.vi"("State(s) in (\"\")"=w185) -> ("States Out"=w184:string)  [unwired: 14 in]
      }
      frame "Data: Initialize" {
        w186 = ""  # Relationships
        w189 = UI_State."Idle"  # State
        w190 = T9 {"Start Ref"=refnum, "Stop Ref"=refnum, "Settings Ref"=refnum, "Exit Ref"=refnum, "Status Ref"=refnum, "Data Ref"=refnum, "Data Source Ref"=refnum}  # UI Refs
        w192 = T7 {"Current VI Reference"=refnum, "Close Panel on Exit?"=FALSE}  # Core
        # "Initialize the shift-register data, here.\n(data names are defined by what you wire into the bundle function)"
        n62 = Bundle("Core"=w192, "UI Refs"=w190, "State"=w189, "Relationships"=w186) -> (w187:T8)  [unwired: 1 in]
        n63 = call <vilib>:"Add State(s) to Queue__JKI_lib_State_Machine.vi"("State(s) in (\"\")"=w194) -> ("States Out"=w193:string)  [unwired: 14 in]
      }
      frame "Data: Set Configuration" {
        n64 = call "Convert API String Arguments to Data.vim"("Reference Type"=w197, "API String"=w198) -> ("error out"=w196:errorcluster, "Data"=w195:T8)  [unwired: 6 in]
      }
      frame "Data: Get Configuration", "Data: Get Internal Data" {
        n65 = call "Query Data as API String Arguments.vim"("Name"=w204, "Cluster Data"=w205) -> ("error"=w203:errorcluster, "API String"=w202:string, "Cluster Data (dup)"=w201:T8)  [unwired: 7 in]
      }
      frame "Data: Cleanup" {
        # "Cleanup any data and references, here.\n(this is called automatically, by the Macro: Exit)"
        n66 = Unbundle By Name(w209) -> ("Core.Current VI Reference"=w212:refnum<vi>)
        n67 = Close Reference(reference=w212, error in (no error)=w211) -> (error out=w210:errorcluster)
        n68 = call <vilib>:"Add State(s) to Queue__JKI_lib_State_Machine.vi"("State(s) in (\"\")"=w214) -> ("States Out"=w213:string)  [unwired: 14 in]
      }
      frame "---------- Events ----------" {
        # "Do not put any code in this frame.\n(It is a separator no-op. You can make a copy of this frame to create a new UI frame)"
        n69 = call <vilib>:"Add State(s) to Queue__JKI_lib_State_Machine.vi"("State(s) in (\"\")"=w219) -> ("States Out"=w218:string)  [unwired: 14 in]
      }
      frame "Events: Register" {
        # "Register message event to break Waiting in Event structure."
        n70 = call <userlib>:"CSM - Get New State Notifier Event.vi"("Name (\"\" to Use UUID)"=w222) -> ("error out"=w220:errorcluster, "New State Notifier Event"=w221:refnum<user-event>)  [unwired: 9 in]
        n71 = register-events(w221) -> (reference out=w223:refnum<event-registration>)  [unwired: 2 in, 1 out]
      }
      frame "Events: Unregister" {
        n72 = Unregister For Events(event registration refnum=w226, error in=w230) -> (error out=w227:errorcluster)
      }
      frame "---------- UI ----------" {
        # "Do not put any code in this frame.\n(It is a separator no-op. You can make a copy of this frame to create a new UI frame)"
        n73 = call <vilib>:"Add State(s) to Queue__JKI_lib_State_Machine.vi"("State(s) in (\"\")"=w235) -> ("States Out"=w234:string)  [unwired: 14 in]
      }
      frame "UI: Initialize" {
        # "Initialize the User Interface, here.\n(this is called automatically, by the Macro: Init)"
        n74 = control-ref of="WaveformGraph"() -> (w242:refnum<vi>)
        n75 = control-ref of="Start"() -> (w246:refnum<vi>)
        n76 = control-ref of="Stop"() -> (w236:refnum<vi>)
        n77 = control-ref of="Settings"() -> (w247:refnum<vi>)
        n78 = control-ref of="Exit"() -> (w248:refnum<vi>)
        n79 = control-ref of="Status"() -> (w243:refnum<vi>)
        n80 = Bundle By Name(cluster=w239, "UI Refs.Start Ref"=w246, "UI Refs.Stop Ref"=w236, "UI Refs.Settings Ref"=w247, "UI Refs.Exit Ref"=w248, "UI Refs.Status Ref"=w243, "UI Refs.Data Ref"=w242) -> (w238:T8)
        n81 = Build Array(w236) -> (w244:refnum<vi>[])
        n82 = Build Array(w246, w248, w247) -> (w245:refnum<vi>[])
        n83 = property on="WaveformGraph" class="WFChart (strict)"("History Data"=waveform(dbl)[][] []) -> ()  [unwired: 2 in, 2 out]
        n84 = call "Set Enable State on Multiple Controls.vi"("Enable?"=TRUE, "Controls"=w245) -> ()  [unwired: 10 in]
        n85 = call "Set Enable State on Multiple Controls.vi"("Enable?"=FALSE, "Controls"=w244) -> ()  [unwired: 10 in]
        n86 = call <vilib>:"Add State(s) to Queue__JKI_lib_State_Machine.vi"("State(s) in (\"\")"=w252) -> ("States Out"=w251:string)  [unwired: 14 in]
      }
      frame "UI: Update When Start" {
        # "Enable: Stop\nDisable: Start, Exit, Settings"
        n87 = Unbundle By Name(w255) -> ("UI Refs.Stop Ref"=w261:refnum<vi>, "UI Refs.Start Ref"=w260:refnum<vi>, "UI Refs.Exit Ref"=w259:refnum<vi>, "UI Refs.Settings Ref"=w258:refnum<vi>, "UI Refs.Data Source Ref"=w254:refnum<vi>)
        n88 = property on="WaveformGraph" class="WFChart (strict)"("History Data"=waveform(dbl)[][] []) -> ()  [unwired: 2 in, 2 out]
        n89 = Build Array(w260, w259, w258, w254) -> (w263:refnum<vi>[])
        n90 = Build Array(w261) -> (w262:refnum<vi>[])
        n91 = call "Set Enable State on Multiple Controls.vi"("Enable?"=TRUE, "Controls"=w262) -> ()  [unwired: 10 in]
        n92 = call "Set Enable State on Multiple Controls.vi"("Enable?"=FALSE, "Controls"=w263) -> ()  [unwired: 10 in]
      }
      frame "UI: Update When Stop" {
        # "Enable: Start, Exit, Settings\nDisable: Stop"
        n93 = Unbundle By Name(w268) -> ("UI Refs.Stop Ref"=w273:refnum<vi>, "UI Refs.Start Ref"=w274:refnum<vi>, "UI Refs.Exit Ref"=w275:refnum<vi>, "UI Refs.Settings Ref"=w276:refnum<vi>, "UI Refs.Data Source Ref"=w267:refnum<vi>)
        n94 = Build Array(w274, w275, w276, w267) -> (w271:refnum<vi>[])
        n95 = Build Array(w273) -> (w272:refnum<vi>[])
        n96 = call "Set Enable State on Multiple Controls.vi"("Enable?"=FALSE, "Controls"=w272) -> ()  [unwired: 10 in]
        n97 = call "Set Enable State on Multiple Controls.vi"("Enable?"=TRUE, "Controls"=w271) -> ()  [unwired: 10 in]
      }
      frame "UI: Cursor Set" {
        # "Argument"
        # "Set and Unset Cursor Busy.\n(Usage: \"UI: Cursor Set >> Busy|Idle\")"
        n98 = disable-structure shown="Default" {
          disable-tunnel: w283 -> [w289 w294]
          disable-tunnel: [w288 w294] -> w282
          disable-tunnel: w281 -> [w287 _]
          frame condition #0 (active) {
            n99 = case shown="\"Busy\"" w287 {
              tunnel: w289 -> [w291 w293]
              tunnel: [w290 w292] -> w288
              frame "Idle", Default {
                n100 = call <vilib>:"Unset Busy.vi"("error in (no error)"=w291) -> ("error out"=w290:errorcluster)  [unwired: 10 in]
              }
              frame "Busy" {
                n101 = call <vilib>:"Set Busy.vi"("error in (no error)"=w293) -> ("error out"=w292:errorcluster)  [unwired: 9 in, 1 out]
              }
            }
          }
          frame condition #1 {
          }
        }
        n102 = call <vilib>:"Add State(s) to Queue__JKI_lib_State_Machine.vi"("State(s) in (\"\")"=w286) -> ("States Out"=w285:string)  [unwired: 14 in]
      }
      frame "UI: Front Panel State" {
        # "Argument"
        # "Set Front Panel Open or Closed\n(Usage: \"UI: Front Panel State >> Open|Close\")"
        n103 = Unbundle By Name(w298) -> ("Core.Current VI Reference"=w297:refnum<vi>)
        n104 = case shown="\"Minimize\", \"Minimized\"" w296 {
          tunnel: w300 -> [w308 w323 w334 w347 w360]
          tunnel: [w310 w324 w336 w349 w362] -> w299
          tunnel: w297 -> [w309 w321 w335 w348 w361]
          frame "Open", "Standard", Default {
            w303 = T2."Standard" ("State")
            n105 = property class="VI"(reference=w309, error in=w308) -> (reference out=w306:refnum<vi>, error out=w307:errorcluster, "FP.State"=w305:T2)
            n106 = Not Equal?(x=w305, y=w303) -> (x != y?=w304:bool)
            n107 = case shown="True" w304 {
              tunnel: [w314 w316] -> w310
              tunnel: w307 -> [w313 w316]
              tunnel: w306 -> [w312 _]
              tunnel: w303 -> [w311 _]
              frame True {
                n108 = invoke class="VI" method="FP.Open"(reference=w312, error in=w313, "Activate"=TRUE, "State"=w311) -> (error out=w314:errorcluster)  [unwired: 1 in, 4 out]
              }
              frame False {
              }
            }
          }
          frame "Close", "Closed" {
            n109 = property class="VI"(reference=w321, error in=w323) -> (reference out=w320:refnum<vi>, error out=w322:errorcluster, "FP.State"=w318:T2)
            n110 = Not Equal?(x=w318, y=T2."Closed" ("Front Panel Window:State")) -> (x != y?=w317:bool)
            n111 = case shown="True" w317 {
              tunnel: [w325 w328] -> w324
              tunnel: w322 -> [w325 w327]
              tunnel: w320 -> [_ w326]
              frame False {
              }
              frame True {
                n112 = invoke class="VI" method="FP.Close"(reference=w326, error in=w327) -> (error out=w328:errorcluster)  [unwired: 1 in, 2 out]
              }
            }
          }
          frame "Hidden", "Hide" {
            w329 = T2."Hidden" ("State")
            n113 = property class="VI"(reference=w335, error in=w334) -> (reference out=w332:refnum<vi>, error out=w333:errorcluster, "FP.State"=w331:T2)
            n114 = Not Equal?(x=w331, y=w329) -> (x != y?=w330:bool)
            n115 = case shown="True" w330 {
              tunnel: [w340 w341] -> w336
              tunnel: w333 -> [w339 w341]
              tunnel: w332 -> [w338 _]
              tunnel: w329 -> [w337 _]
              frame True {
                n116 = invoke class="VI" method="FP.Open"(reference=w338, error in=w339, "State"=w337) -> (error out=w340:errorcluster)  [unwired: 2 in, 4 out]
              }
              frame False {
              }
            }
          }
          frame "Minimize", "Minimized" {
            w342 = T2."Minimized" ("State")
            n117 = property class="VI"(reference=w348, error in=w347) -> (reference out=w345:refnum<vi>, error out=w346:errorcluster, "FP.State"=w344:T2)
            n118 = Not Equal?(x=w344, y=w342) -> (x != y?=w343:bool)
            n119 = case shown="True" w343 {
              tunnel: [w353 w354] -> w349
              tunnel: w346 -> [w352 w354]
              tunnel: w345 -> [w351 _]
              tunnel: w342 -> [w350 _]
              frame True {
                n120 = invoke class="VI" method="FP.Open"(reference=w351, error in=w352, "State"=w350) -> (error out=w353:errorcluster)  [unwired: 2 in, 4 out]
              }
              frame False {
              }
            }
          }
          frame "Maximize", "Maximized" {
            w355 = T2."Maximized" ("State")
            n121 = property class="VI"(reference=w361, error in=w360) -> (reference out=w358:refnum<vi>, error out=w359:errorcluster, "FP.State"=w357:T2)
            n122 = Not Equal?(x=w357, y=w355) -> (x != y?=w356:bool)
            n123 = case shown="True" w356 {
              tunnel: [w366 w367] -> w362
              tunnel: w359 -> [w365 w367]
              tunnel: w358 -> [w364 _]
              tunnel: w355 -> [w363 _]
              frame True {
                n124 = invoke class="VI" method="FP.Open"(reference=w364, error in=w365, "State"=w363) -> (error out=w366:errorcluster)  [unwired: 2 in, 4 out]
              }
              frame False {
              }
            }
          }
        }
        n125 = call <vilib>:"Add State(s) to Queue__JKI_lib_State_Machine.vi"("State(s) in (\"\")"=w302) -> ("States Out"=w301:string)  [unwired: 14 in]
      }
      frame "UI: Change Waveform Graph Legend Num" {
        n126 = Unbundle By Name(w374) -> ("UI Refs.Data Ref"=w373:refnum<vi>)
        n127 = call "Convert API String Arguments to Data.vim"("Reference Type"=u32 0 ("Legend:Number of Rows"), "API String"=w371) -> ("error out"=w369:errorcluster, "Data"=w372:u32)  [unwired: 6 in]
        n128 = property class="WFChart (strict)"(reference=w373, error in=w369, "LegNumRows"=w372) -> (error out=w368:errorcluster)  [unwired: 1 out]
      }
      frame "UI: Update Waveform Graph" {
        n129 = call "CSM - Convert Argument to MassData.vim"("Type"=waveform(dbl)[] [] ("Data"), "MassData Argument"=w389) -> ("error out"=w387:errorcluster, "Data"=w383:waveform(dbl)[])  [unwired: 6 in]
        "WaveformGraph" <- w383
        n130 = Array Size(array=w383) -> (size(s)=w380:i32)
        n131 = feedback-in #1(w380) -> ()
        n132 = feedback #1(0) -> (w381:i32)
        n133 = Not Equal?(x=w380, y=w381) -> (x != y?=w377:bool)
        n134 = Format Into String(w380) -> (resulting string=w382:string)  [unwired: 3 in, 1 out]
        n135 = call <vilib>:"Build State String with Arguments__JKI_lib_State_Machine.vi"("Arguments (\"\")"=w382, "State"="UI: Change Waveform Graph Legend Num") -> ("State with Arguments"=w378:string)  [unwired: 4 in]
        n136 = call-poly <userlib>:"Add State(s) to Queue By BOOL++.vi"("TRUE (\"\")"=w378, "Condition"=w377, "State Queue (\"\")"=w385) -> ("Remaining States"=w386:string)  [unwired: 8 in]
      }
      frame "---------- Macro ----------" {
        n137 = call <vilib>:"Add State(s) to Queue__JKI_lib_State_Machine.vi"("State(s) in (\"\")"=w396) -> ("States Out"=w395:string)  [unwired: 14 in]
      }
      frame "Macro: Initialize" {
        w397 = "Data: Initialize\nInitialize Core Data\nEvents: Register\nUI: Initialize\nUI: Front Panel State >> Open\nUI: Change Waveform Graph Legend Num >> 1\nDO: Update Status >> Ready...\n\n//Permanent registrations\nAcquired Waveform@Acquisition >> API: Log@Logging -><register>\nAcquired Waveform@Acquisition >> UI: Update Waveform Graph -><register>"  # Data: Initialize Initialize Core Data Events: Register UI: Initialize UI: Front Panel State >> Open UI: Change Waveform Graph Legend Num >> 1 DO: Update Status >> Ready...  //Permanent registrations Acquired Waveform@Acquisition >> API: Log@Logging -><register> Acquired Waveform@Acquisition >> UI: Update Waveform Graph -><register>
        # "Initialization Macro\n(This is called once, when the VI starts)"
        n138 = call <userlib>:"CSM - Populate Configuration Variables.vi"("String with INI-Variable"=w397) -> ("String"=w398:string)  [unwired: 7 in, 1 out]
        n139 = call <vilib>:"Add State(s) to Queue__JKI_lib_State_Machine.vi"("State(s) in Front (\"\")"=w398, "State(s) in (\"\")"=w403) -> ("States Out"=w402:string)  [unwired: 13 in]
      }
      frame "Macro: Start" {
        n140 = Bundle By Name(cluster=w408, "State"=UI_State."Acquiring and Logging" ("UI State")) -> (w407:T8)
        n141 = call <vilib>:"Add State(s) to Queue__JKI_lib_State_Machine.vi"("State(s) in Front (\"\")"="//Local States\nDO: Update Status >> Acquiring and Logging...\nUI: Update When Start\n\n//Send Message to Other CSM Modules\nAPI: Start -@ Logging\nAPI: Start ->| Acquisition" ("State(s) in Front (\"\")"), "State(s) in (\"\")"=w405) -> ("States Out"=w406:string)  [unwired: 13 in]
      }
      frame "Macro: Stop" {
        n142 = Unbundle By Name(w412) -> ("State"=w414:T4)
        n143 = case shown="Default" w414 {
          selector: w414 -> [w421 _]
          tunnel: [w421 UI_State."Waiting for Stop" ("UI State")] -> w413
          frame "Waiting for Exit" {
          }
          frame Default {
          }
        }
        n144 = Bundle By Name(cluster=w412, "State"=w413) -> (w418:T8)
        n145 = call <vilib>:"Add State(s) to Queue__JKI_lib_State_Machine.vi"("State(s) in Front (\"\")"="//Local States\nDO: Update Status >> Stopping...\nUI: Update When Stop\n\n//Send Message to Other CSM Modules\nAPI: Stop -@ Acquisition\nAPI: Stop -@ Logging\n" ("State(s) in Front (\"\")"), "State(s) in (\"\")"=w416) -> ("States Out"=w417:string)  [unwired: 13 in]
      }
      frame "Macro: Exit" {
        w430 = "//UI: Front Panel State >> Close"  # //UI: Front Panel State >> Close
        w427 = "//Permanent registrations\nAcquired Waveform@Acquisition >> API: Log@Logging -><unregister>\nAcquired Waveform@Acquisition >> UI: Update Waveform Graph -><unregister>\n\nData: Cleanup\nEvents: Unregister\nExit"  # //Permanent registrations Acquired Waveform@Acquisition >> API: Log@Logging -><unregister> Acquired Waveform@Acquisition >> UI: Update Waveform Graph -><unregister>  Data: Cleanup Events: Unregister Exit
        # "Exit Macro\n(This is called once, when the VI exits)"
        n146 = Unbundle By Name(w432) -> ("Core.Close Panel on Exit?"=w431:bool)
        n147 = disable-structure shown="Disabled" {
          disable-tunnel: [w435 w451 w453] -> w424
          disable-tunnel: w423 -> [_ w446 _]
          frame Disabled {
            w442 = "Macro: Exit -@ Acquisition\nMacro: Exit -@ Logging"  # Macro: Exit -@ Acquisition Macro: Exit -@ Logging
            n148 = call <userlib>:"CSM - Module Status.vi"("CSM Name"="Algorithm") -> ("#Nodes"=w438:i32, "CSM Name (Dup)"=w440:string)  [unwired: 6 in, 3 out]
            n149 = for {
              N: w438 -> [_]
              tunnel: w440 -> [w445]
              tunnel: "Macro: Exit" -> [w444]
              tunnel: [w443] -> w436 mode=indexing
              n150 = call-poly <userlib>:"Build Message with Arguments++.vi"("State With Arguments"=w444, "Target Module (\"\")"=w445) -> ("CSM Message String"=w443:string)  [unwired: 13 in]
            }
            n151 = Build Array (concatenate)(w442, w436) -> (w437:string[])
            n152 = call <userlib>:"CSM - Compact Multiple States.vi"("Multiple States"=w437) -> ("States"=w435:string)  [unwired: 9 in]
          }
          frame Enabled {
            # "#NOTE\nHelper VI is equivalent to other case"
            n153 = call <userlib>:"CSM - List Modules.vi"() -> ("Module Names"=w448:string[])  [unwired: 10 in, 1 out]
            n154 = Search 1D Array(1D array=w448, element=w446) -> (index of element=w449:i32)  [unwired: 1 in]
            n155 = Delete From Array(array=w448, index=w449) -> (array with subset deleted=w447:string[])  [unwired: 1 in, 1 out]
            n156 = call <userlib>:"CSM - Build Exit Messages of CSMs.vi"("State With Arguments (\"Macro: Exit“)"="Macro: Exit" ("State with Arguments(\"Macro: Exit“)"), "CSMs"=w447) -> ("States"=w451:string)  [unwired: 13 in]
          }
          frame Disabled {
            # "#NOTE\nHelper VI is equivalent to other case"
            n157 = call <userlib>:"CSM - Build Exit Messages of CSMs.vi"("State With Arguments (\"Macro: Exit“)"="Macro: Exit" ("State with Arguments(\"Macro: Exit“)"), "CSMs"=string[] ["Acquisition", "Logging", "Algorithm"]) -> ("States"=w453:string)  [unwired: 13 in]
          }
        }
        n158 = Select(t=w430, s=w431, f="") -> (s? t:f=w428:string)
        n159 = call <vilib>:"Add State(s) to Queue__JKI_lib_State_Machine.vi"("State(s) in Front (\"\")"=w424, "State(s) in (\"\")"=w428, "State(s) at Back (\"\")"=w427) -> ("States Out"=w426:string)  [unwired: 12 in]
        n160 = call <vilib>:"Add State(s) to Queue__JKI_lib_State_Machine.vi"("State(s) in Front (\"\")"=w426, "State(s) in (\"\")"=w434) -> ("States Out"=w433:string)  [unwired: 13 in]
      }
      frame "---------- DoSth ----------" {
        n161 = call <vilib>:"Add State(s) to Queue__JKI_lib_State_Machine.vi"("State(s) in (\"\")"=w459) -> ("States Out"=w458:string)  [unwired: 14 in]
      }
      frame "Do: Update Status" {
        n162 = call <vilib>:"Add State(s) to Queue__JKI_lib_State_Machine.vi"("State(s) in (\"\")"=w465) -> ("States Out"=w464:string)  [unwired: 14 in]
        "Status" <- w460
      }
      frame "Do: Launch Settings Dialog" {
        # "Your code here.\n(You can make a copy of, or modify, this frame)"
        n163 = call <userlib>:"CSM - Check If Module Exists.vi"("CSM Name"="Acquisition" ("Name(\"\" to use uuid)")) -> ("error out"=w472:errorcluster, "Exist?"=w468:bool, "CSM Name (Dup)"=w470:string)  [unwired: 8 in]
        n164 = case shown="True" w468 {
          tunnel: w472 -> [w480 w492]
          tunnel: w470 -> [w476 w491]
          tunnel: w469 -> [_ w490]
          tunnel: [w479 w489] -> w467
          frame False {
            n165 = Format Into String(format string="Cannot Find the CSM which named %s !!!", w476) -> (resulting string=w475:string)  [unwired: 2 in, 1 out]
            n166 = Bundle By Name(cluster=w480, "status"=TRUE, "source"=w475) -> (w479:errorcluster)
          }
          frame True {
            w484 = T2."Standard" ("State")
            n167 = call <userlib>:"CSM - Module VI Reference.vi"("Current Module (\"\" to Generate an ID)"=w490, "error in (no error)"=w492, "Force? (F)"=TRUE ("force?(F)"), "CSM Name"=w491) -> ("error out"=w482:errorcluster, "CSM Module VIRef"=w483:refnum<vi>)  [unwired: 6 in]
            n168 = property class="VI"(reference=w483, error in=w482) -> (reference out=w487:refnum<vi>, error out=w488:errorcluster, "FP.State"=w486:T2)
            n169 = Not Equal?(x=w486, y=w484) -> (x != y?=w485:bool)
            n170 = case shown="True" w485 {
              tunnel: [w499 w501] -> w489
              tunnel: w488 -> [w494 w501]
              tunnel: w487 -> [w493 _]
              tunnel: w484 -> [w498 _]
              frame True {
                n171 = property class="VI"(reference=w493, error in=w494, "FP.Behavior"=T5."Modal" ("Front Panel Window:Behavior")) -> (reference out=w496:refnum<vi>, error out=w497:errorcluster)
                n172 = invoke class="VI" method="FP.Open"(reference=w496, error in=w497, "Activate"=TRUE, "State"=w498) -> (error out=w499:errorcluster)  [unwired: 1 in, 4 out]
              }
              frame False {
              }
            }
          }
        }
      }
      frame "Do: Confirm Quit" {
        n173 = Unbundle By Name(w506) -> ("State"=w509:T4)
        n174 = case shown="Default" w509 {
          tunnel: [UI_State."Idle" ("UI State") w518] -> w508
          tunnel: w506 -> [w513 w517]
          tunnel: [w513 w516] -> w507
          tunnel: [TRUE w515] -> w502
          frame Default {
          }
          frame "Acquiring and Logging" {
            n175 = Two Button Dialog(message="Are you sure you want to quit while the acquisition is running?" ("Confirm Quit Message"), 1:"No" ("No"), 2:"Yes" ("Yes")) -> (T button?=w519:bool)
            n176 = case shown="False" w519 {
              tunnel: [UI_State."Acquiring and Logging" ("UI State") UI_State."Waiting for Exit" ("UI State")] -> w518
              tunnel: w517 -> [w523 w526]
              tunnel: [w523 w526] -> w516
              tunnel: [_ TRUE] -> w515
              frame False {
                # "User did not want to quit."
              }
              frame True {
              }
            }
          }
        }
        n177 = Bundle By Name(cluster=w507, "State"=w508) -> (w505:T8)
        n178 = call-poly <userlib>:"Add State(s) to Queue By BOOL++.vi"("TRUE (\"\")"="Macro: Exit", "Condition"=w502, "State Queue (\"\")"=w511) -> ("Remaining States"=w504:string)  [unwired: 8 in]
      }
    }
  }
  n179 = call <userlib>:"CSM - Sync Configuration Variables to File.vi"("All Temp Variable to Default Ini(F)"=TRUE, "error in (no error)"=w2) -> ("error out"=w1:errorcluster)  [unwired: 7 in]
  n180 = disable-structure shown="RUN_TIME_ENGINE==True" {
    disable-tunnel: w1 -> [_ _]
    frame condition #0 (active) {
    }
    frame condition #1 {
      n181 = Quit LabVIEW(quit? (T)=TRUE) -> ()
    }
  }
